vi "FTW-Connector-Connect.vi"(0 "FTW Actor Connector Type":refnum<class "FTW-ActorConnector.lvclass">, 5 "Instance Inbox Address":string, 11 "error in":errorcluster) -> (4 "FTW Actor Connector":refnum<class "FTW-ActorConnector.lvclass">, 15 "error out":errorcluster)   [LabVIEW 2013, in "FTW-ActorConnector.lvclass"]
uses:
  FTW-ActorConnector.lvclass
  FTW-ActorConnector.lvclass/FTW-ActorConnector.ctl
  Request/FTW-Request.lvclass
panel:
  # "Inputs"
  # "Outputs"
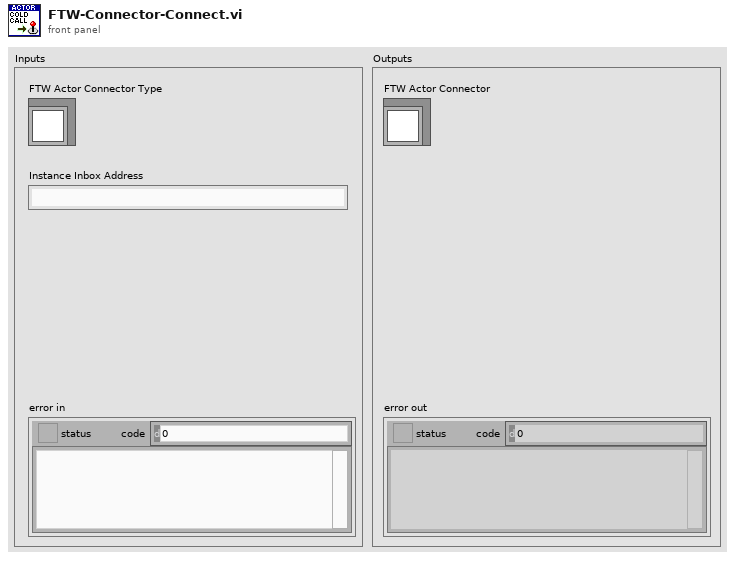
[diagram p1: front panel]
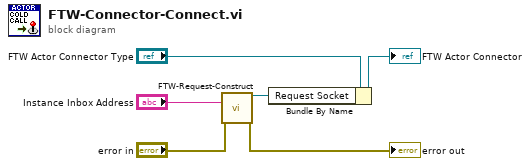
[diagram p0: block diagram]
diagram:
  n1 = call "FTW-Request-Construct.vi"("Server Address"="Instance Inbox Address", "error in"="error in") -> ("FTW-Request Out"=w1:refnum<class "FTW-Request.lvclass">, "error out"=→"error out":errorcluster)  [unwired: 12 in]
  n2 = Bundle By Name(cluster="FTW Actor Connector Type", "Request Socket"=w1) -> (→"FTW Actor Connector":refnum<class "FTW-ActorConnector.lvclass">)
